vi "Set Shooter RPM.vi"(6 "Key Shot":bool, 8 "Open Loop":bool, 9 "Increment":bool, 10 "Decrement":bool, 11 "Shooter Enabled":bool) -> ()   [LabVIEW 2011]
uses:
  System Set Points and States.vi
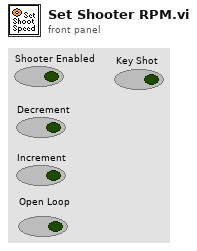
[diagram p1: front panel]
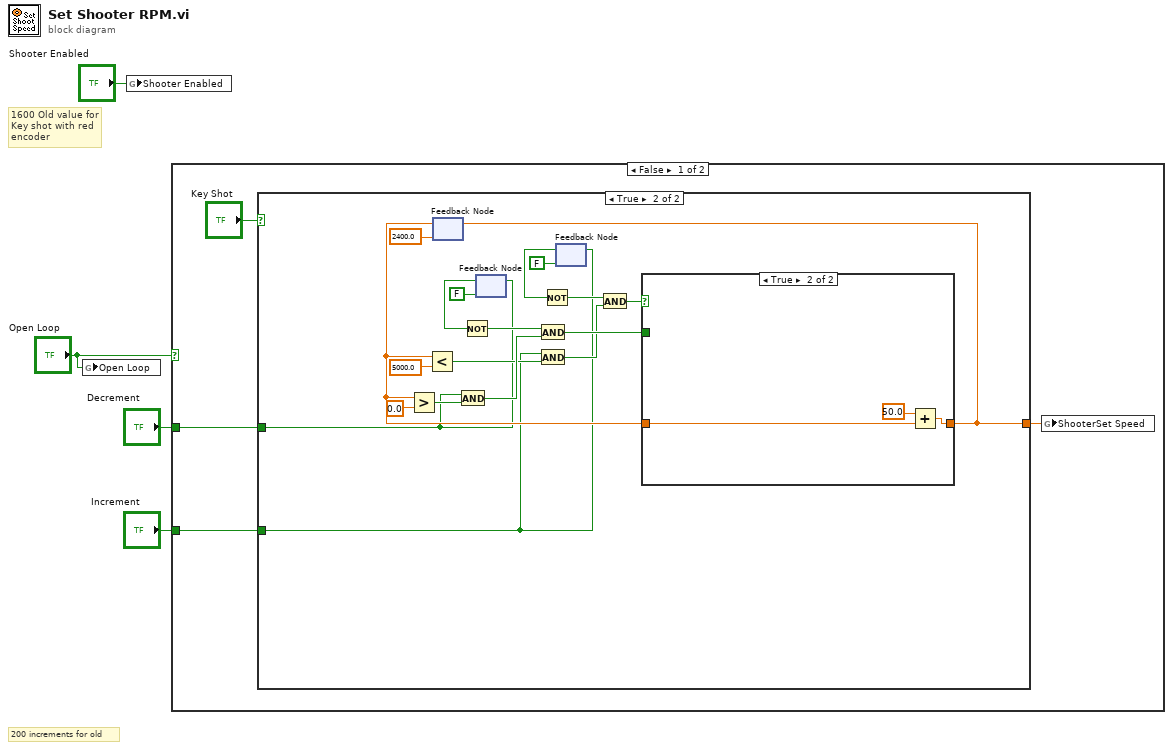
[diagram p0: block diagram]
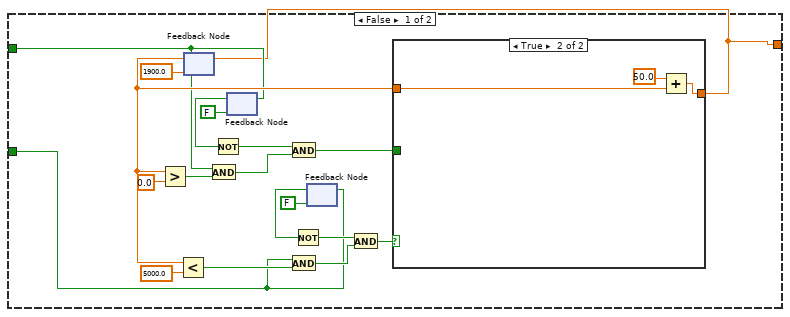
[diagram p2: hidden frame]
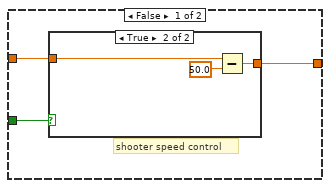
[diagram p3: hidden frame]
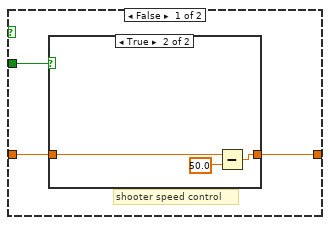
[diagram p5: hidden frame]
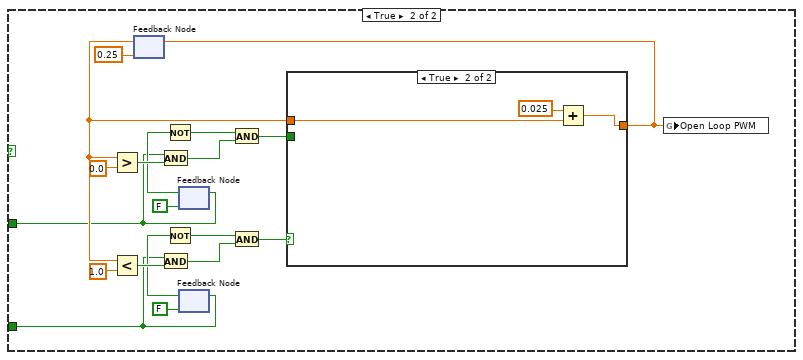
[diagram p7: hidden frame]
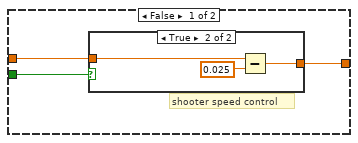
[diagram p8: hidden frame]
diagram:
  # "200 increments for old"
  # "1600 Old value for\nKey shot with red\nencoder"
  n1 = global write "System Set Points and States.vi" "Open Loop"("Open Loop") -> ()
  n2 = global write "System Set Points and States.vi" "Shooter Enabled"("Shooter Enabled") -> ()
  n3 = case shown="False" "Open Loop" {
    tunnel: "Decrement" -> [w8 w69]
    tunnel: "Increment" -> [w7 w68]
    frame False {
      n4 = case shown="True" "Key Shot" {
        tunnel: w8 -> [w11 w40]
        tunnel: w7 -> [w10 w39]
        tunnel: [w9 w38] -> w6
        frame False {
          n5 = feedback #1(1900.0) -> (w14:dbl)
          n6 = Greater?(x=w14, y=0.0) -> (0:w12:bool)
          n7 = Less?(x=w14, y=5000.0) -> (x < y?=w15:bool)
          n8 = And(x=w11, y=w12) -> (x .and. y?=w21:bool)
          n9 = feedback #2(FALSE) -> (w25:bool)
          n10 = Not(x=w25) -> (.not. x?=w26:bool)
          n11 = feedback-in #2(w11) -> ()
          n12 = And(x=w26, y=w21) -> (x .and. y?=w22:bool)
          n13 = And(x=w10, y=w15) -> (x .and. y?=w18:bool)
          n14 = feedback #3(FALSE) -> (w23:bool)
          n15 = Not(x=w23) -> (.not. x?=w24:bool)
          n16 = feedback-in #3(w10) -> ()
          n17 = And(x=w24, y=w18) -> (x .and. y?=w19:bool)
          n18 = case shown="True" w19 {
            tunnel: w22 -> [w30 _]
            tunnel: w14 -> [w29 w37]
            tunnel: [w28 w35] -> w9
            frame False {
              # "shooter speed control"
              n19 = case shown="True" w30 {
                tunnel: w29 -> [w31 w34]
                tunnel: [w31 w32] -> w28
                frame False {
                }
                frame True {
                  n20 = Subtract(x=w34, y=50.0) -> (x-y=w32:dbl)
                }
              }
            }
            frame True {
              n21 = Add(x=50.0, y=w37) -> (x+y=w35:dbl)
            }
          }
          n22 = feedback-in #1(w9) -> ()
        }
        frame True {
          n23 = feedback #4(2400.0) -> (w43:dbl)
          n24 = Greater?(x=w43, y=0.0) -> (0:w41:bool)
          n25 = Less?(x=w43, y=5000.0) -> (x < y?=w44:bool)
          n26 = And(x=w40, y=w41) -> (x .and. y?=w50:bool)
          n27 = feedback #5(FALSE) -> (w54:bool)
          n28 = Not(x=w54) -> (.not. x?=w55:bool)
          n29 = feedback-in #5(w40) -> ()
          n30 = And(x=w55, y=w50) -> (x .and. y?=w51:bool)
          n31 = And(x=w39, y=w44) -> (x .and. y?=w47:bool)
          n32 = feedback #6(FALSE) -> (w52:bool)
          n33 = Not(x=w52) -> (.not. x?=w53:bool)
          n34 = feedback-in #6(w39) -> ()
          n35 = And(x=w53, y=w47) -> (x .and. y?=w48:bool)
          n36 = case shown="True" w48 {
            tunnel: w51 -> [w59 _]
            tunnel: w43 -> [w58 w66]
            tunnel: [w57 w64] -> w38
            frame False {
              # "shooter speed control"
              n37 = case shown="True" w59 {
                tunnel: w58 -> [w60 w63]
                tunnel: [w60 w61] -> w57
                frame False {
                }
                frame True {
                  n38 = Subtract(x=w63, y=50.0) -> (x-y=w61:dbl)
                }
              }
            }
            frame True {
              n39 = Add(x=50.0, y=w66) -> (x+y=w64:dbl)
            }
          }
          n40 = feedback-in #4(w38) -> ()
        }
      }
      n41 = global write "System Set Points and States.vi" "ShooterSet Speed"(w6) -> ()
    }
    frame True {
      n42 = feedback #7(0.25) -> (w72:dbl)
      n43 = Greater?(x=w72, y=0.0) -> (0:w85:bool)
      n44 = Less?(x=w72, y=1.0) -> (x < y?=w83:bool)
      n45 = And(x=w69, y=w85) -> (x .and. y?=w78:bool)
      n46 = And(x=w68, y=w83) -> (x .and. y?=w80:bool)
      n47 = feedback #8(FALSE) -> (w75:bool)
      n48 = Not(x=w75) -> (.not. x?=w74:bool)
      n49 = feedback-in #8(w69) -> ()
      n50 = feedback #9(FALSE) -> (w77:bool)
      n51 = Not(x=w77) -> (.not. x?=w76:bool)
      n52 = feedback-in #9(w68) -> ()
      n53 = And(x=w74, y=w78) -> (x .and. y?=w71:bool)
      n54 = And(x=w76, y=w80) -> (x .and. y?=w70:bool)
      n55 = case shown="True" w70 {
        tunnel: w71 -> [w88 _]
        tunnel: w72 -> [w87 w95]
        tunnel: [w86 w93] -> w67
        frame False {
          # "shooter speed control"
          n56 = case shown="True" w88 {
            tunnel: w87 -> [w89 w92]
            tunnel: [w89 w90] -> w86
            frame False {
            }
            frame True {
              n57 = Subtract(x=w92, y=0.025) -> (x-y=w90:dbl)
            }
          }
        }
        frame True {
          n58 = Add(x=0.025, y=w95) -> (x+y=w93:dbl)
        }
      }
      n59 = feedback-in #7(w67) -> ()
      n60 = global write "System Set Points and States.vi" "Open Loop PWM"(w67) -> ()
    }
  }
